vi "HardwareInitialize.vi"(8 "Error In":errorcluster, 11 "Executable Configuration":T1) -> (0 "Error Out":errorcluster, 3 "Keithley 2602 Out":refnum<visa-resource-name>)   [LabVIEW 2012]
uses:
  ExecutableConfiguration.ctl
  driver/Public/Controls/DisplayScreen.ctl
  driver/Keithley-2602.lvlib
  libs/LV-Utilities/LV-Utilities.lvlib
panel:
  out "Found?":bool
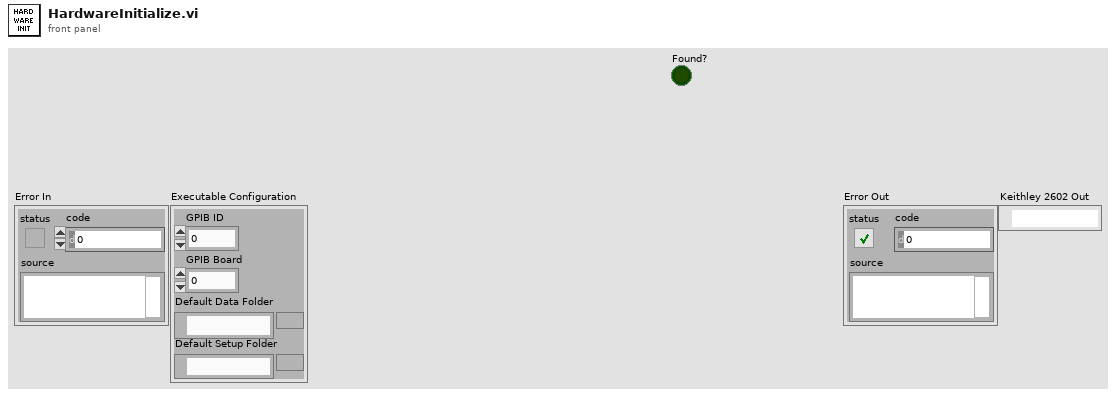
[diagram p1: front panel]
types:
  T1 = typedef "ExecutableConfiguration.ctl" = cluster{"GPIB ID":u8, "GPIB Board":u8, "Default Data Folder":path, "Default Setup Folder":path}
  T2 = typedef "Keithley-2602.lvlib/DisplayScreen.ctl" = enum16{"SMU A", "SMU B", "Both", "User"}
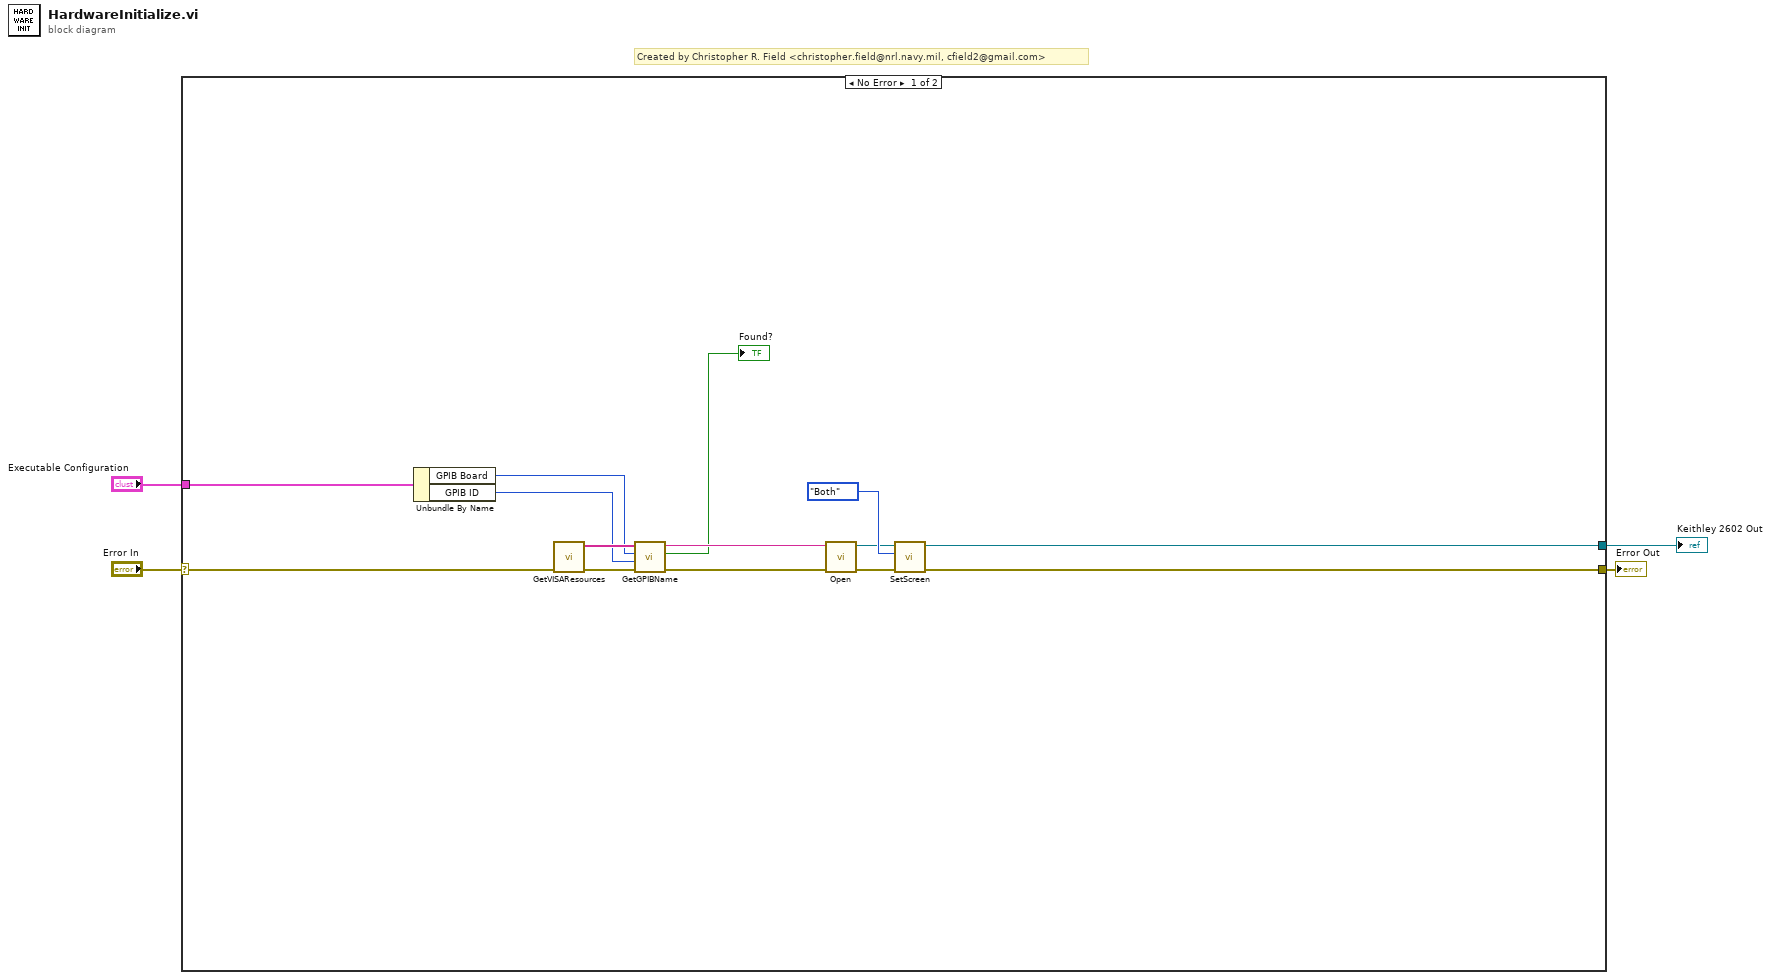
[diagram p0: block diagram]
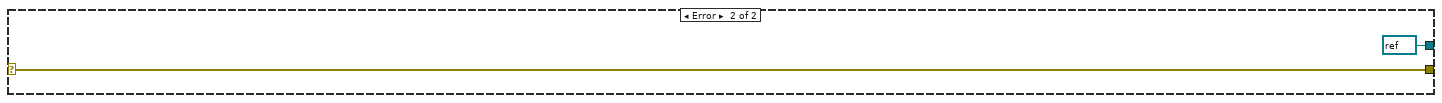
[diagram p2: hidden frame]
diagram:
  # "Created by Christopher R. Field <christopher.field@nrl.navy.mil, cfield2@gmail.com>"
  n1 = case shown="No Error" "Error In" {
    selector: "Error In" -> [w11 w20]
    tunnel: [w10 w20] -> w3
    tunnel: [w9 refnum<visa-resource-name> refnum ("Keithley 2602 Out")] -> w2
    tunnel: "Executable Configuration" -> [w6 _]
    frame No Error {
      n2 = Unbundle By Name(w6) -> ("GPIB Board"=w8:u8, "GPIB ID"=w7:u8)
      n3 = call "GetVISAResources.vi"("Error In"=w11) -> ("Error Out"=w17:errorcluster, "VISA Resources"=w18:string[])  [unwired: 9 in]
      n4 = call "GetGPIBName.vi"("Error In"=w17, "GPIB ID"=w7, "GPIB Board"=w8, "VISA Resource List"=w18) -> ("Error Out"=w15:errorcluster, "Found?"=→"Found?":bool, "VISA GPIB Resource Name"=w16:string)  [unwired: 5 in]
      n5 = call "Open.vi"("Error In"=w15, "Keithley 2602 In"=w16) -> ("Error Out"=w12:errorcluster, "Keithley 2602 Out"=w13:refnum<visa-resource-name>)  [unwired: 8 in]
      n6 = call "SetScreen.vi"("Error In"=w12, "Display Screen"=DisplayScreen."Both", "Keithley 2602 In"=w13) -> ("Error Out"=w10:errorcluster, "Keithley 2602 Out"=w9:refnum<visa-resource-name>)  [unwired: 7 in]
    }
    frame Error {
    }
  }
  "Error Out" <- w3
  "Keithley 2602 Out" <- w2
